vi "2810A Open Ref.vi"(8 "error in":errorcluster, 11 "JSONCluster":T1) -> (0 "error out":errorcluster, 3 "IVI Refnum out":refnum<k15>)   [LabVIEW 2019, in "SupportVIs.lvlib"]
uses:
  SupportVIs.lvlib
  JSONCluster.ctl
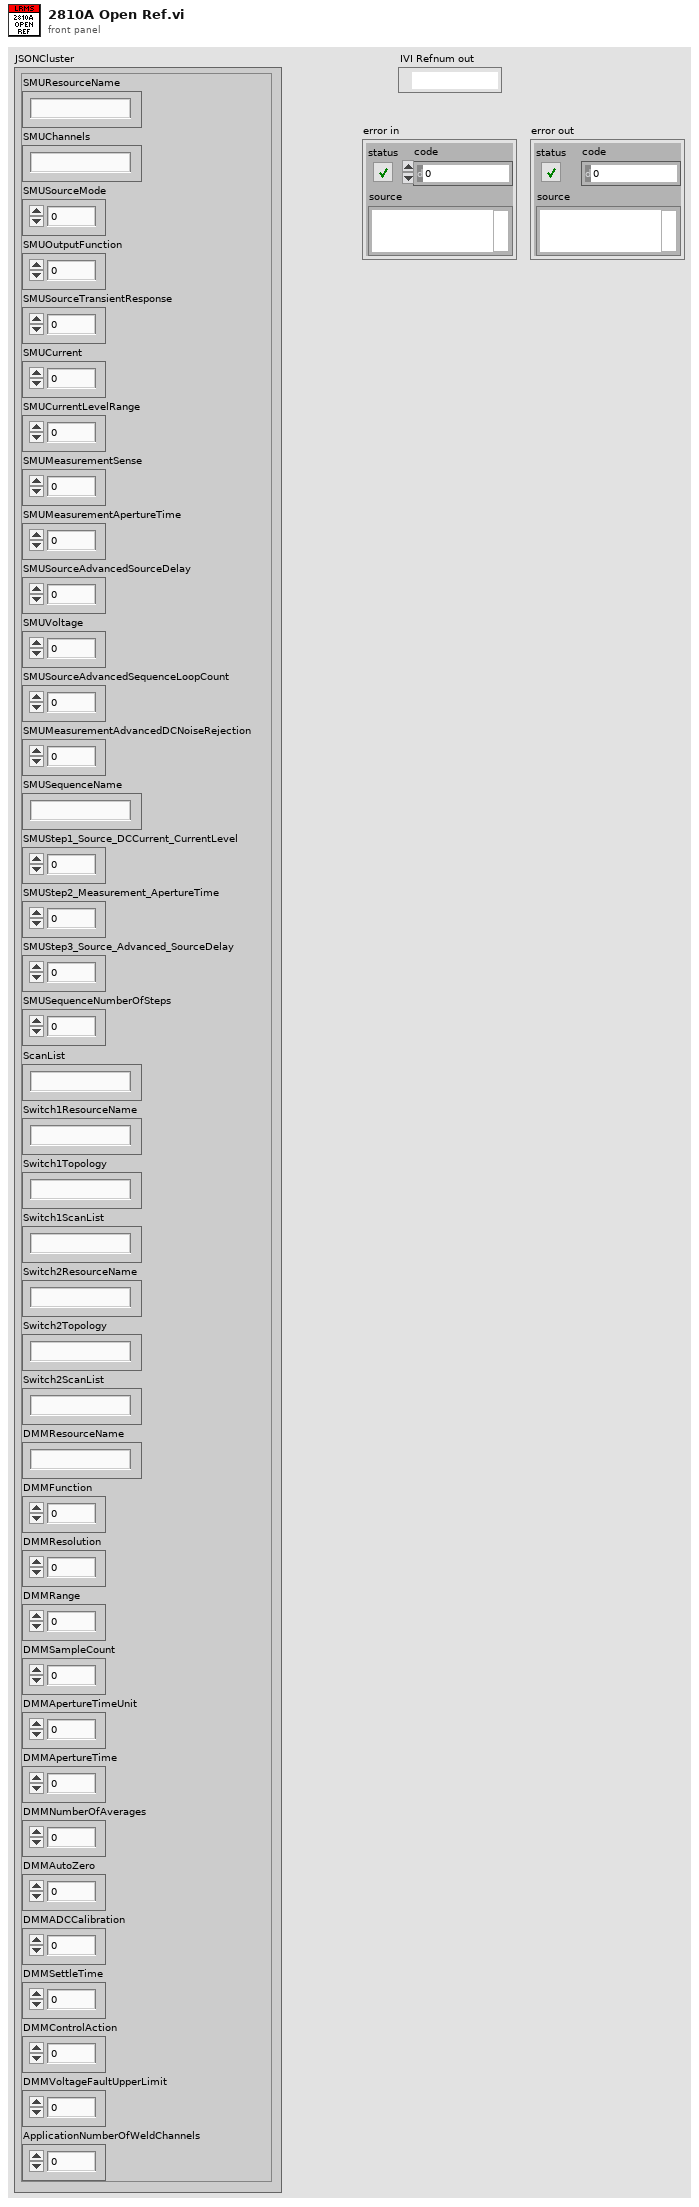
[diagram p1: front panel]
types:
  T1 = typedef "JSONCluster.ctl" = cluster{"SMUResourceName":string, "SMUChannels":string, "SMUSourceMode":i32, "SMUOutputFunction":i32, "SMUSourceTransientResponse":i32, "SMUCurrent":dbl, "SMUCurrentLevelRange":dbl, "SMUMeasurementSense":i32, "SMUMeasurementApertureTime":dbl, "SMUSourceAdvancedSourceDelay":dbl, "SMUVoltage":dbl, "SMUSourceAdvancedSequenceLoopCount":i32, "SMUMeasurementAdvancedDCNoiseRejection":i32, "SMUSequenceName":string, "SMUStep1_Source_DCCurrent_CurrentLevel":i32, "SMUStep2_Measurement_ApertureTime":i32, "SMUStep3_Source_Advanced_SourceDelay":i32, "SMUSequenceNumberOfSteps":i32, "ScanList":string, "Switch1ResourceName":string, "Switch1Topology":string, "Switch1ScanList":string, "Switch2ResourceName":string, "Switch2Topology":string, "Switch2ScanList":string, "DMMResourceName":string, "DMMFunction":i32, "DMMResolution":dbl, "DMMRange":dbl, "DMMSampleCount":i32, "DMMApertureTimeUnit":i32, "DMMApertureTime":dbl, "DMMNumberOfAverages":i32, "DMMAutoZero":i32, "DMMADCCalibration":i32, "DMMSettleTime":dbl, "DMMControlAction":i32, "DMMVoltageFaultUpperLimit":dbl, "ApplicationNumberOfWeldChannels":i32}
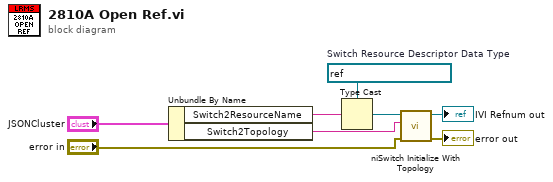
[diagram p0: block diagram]
diagram:
  w4 = refnum<k15> "SwitchBlock1Dev1"  # Switch Resource Descriptor Data Type
  n1 = Unbundle By Name("JSONCluster") -> ("Switch2ResourceName"=w5:string, "Switch2Topology"=w2:string)
  n2 = Type Cast(type=w4, x=w5) -> (*(type *) &x=w3:refnum<k15>)
  n3 = call <instrlib>:"niSwitch Initialize With Topology.vi"("error in (no error)"="error in", "topology name"=w2, "resource name"=w3) -> ("error out"=→"error out":errorcluster, "instrument handle out"=→"IVI Refnum out":refnum<k15>)  [unwired: 2 in, 5 out]
